vi "www template header.vi"(8 "error in (no error)":errorcluster, 11 "Template Content (\"\")":string) -> (0 "error out":errorcluster, 3 "Template Content":string)   [LabVIEW 2011]
uses:
  ITK EXT/utils/strutil.llb/Case Matching.ctl
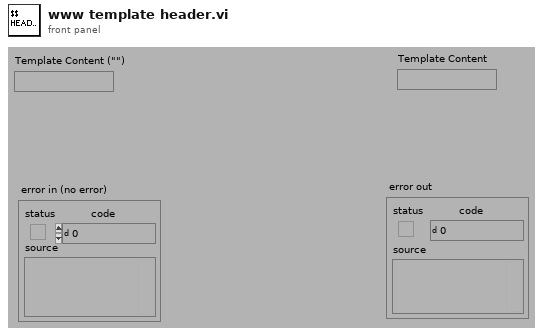
[diagram p1: front panel]
types:
  T1 = typedef "Keyed Array.ctl" = cluster{"keys":string[], "values":string[]}
  T2 = typedef "Case Matching.ctl" = enum16{"a != A", "a == A", "system"}
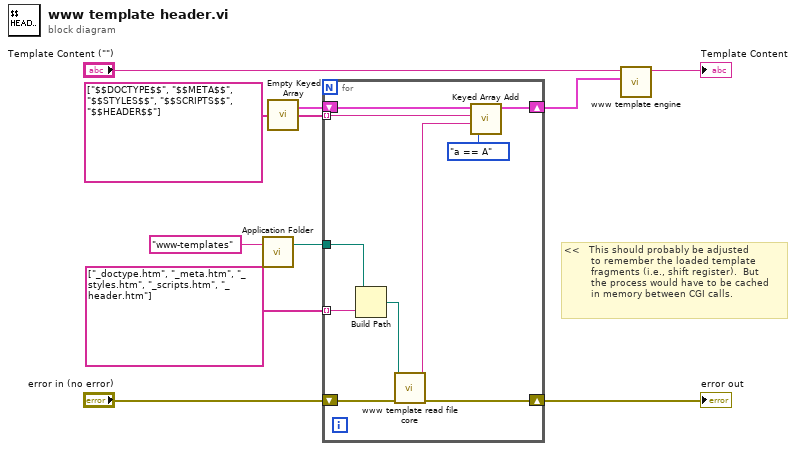
[diagram p0: block diagram]
diagram:
  # "<<   This should probably be adjusted\n         to remember the loaded template\n         fragments (i.e., shift register).  But\n         the process would have to be cached\n         in memory between CGI calls."
  n1 = call "Application Folder.vi"("Relative Path (\"\" - Folder)"="www-templates" ("name or relative path")) -> ("Application Folder"=w1:path)  [unwired: 2 in]
  n2 = call "Empty Keyed Array.vi"() -> ("empty keyed array"=w6:T1)  [unwired: 3 out]
  n3 = for {
    tunnel: w1 -> [w20]
    tunnel: string[] ["_doctype.htm", "_meta.htm", "_styles.htm", "_scripts.htm", "_header.htm"] -> [w19] mode=indexing
    shift-right: [w16] -> w4
    shift-left: "error in (no error)" -> [w17]
    shift-right: [w15] -> w7
    shift-left: w6 -> [w14]
    tunnel: string[] ["$$DOCTYPE$$", "$$META$$", "$$STYLES$$", "$$SCRIPTS$$", "$$HEADER$$"] -> [w13] mode=indexing
    n4 = Build Path(base path=w20, name or relative path=w19) -> (appended path=w18:path)
    n5 = call "www template read file core.vi"("error in (no error)"=w17, "Path"=w18) -> ("error out"=w16:errorcluster, "File Content"=w11:string)  [unwired: 8 out]
    n6 = call "Keyed Array Add.vi"("case matching (sensitive)"=Case_Matching."a == A", "value"=w11, "key"=w13, "array in"=w14) -> ("array out"=w15:T1)  [unwired: 3 out]
  }
  "error out" <- w4
  n7 = call "www template engine.vi"("Template Dictionary (empty)"=w7, "Template String (\"\")"="Template Content (\"\")") -> ("Template String out"=→"Template Content":string)  [unwired: 1 in, 8 out]
